vi "control_posicion_DAQ.vi"() -> ()   [LabVIEW 2025]
uses:
  <vilib>/addons/control/pid/pid.llb/PID (DBL).vi
  <vilib>/addons/control/pid/NI_PID_pid.lvlib
panel:
  out "Error":dynamicdata(graph)
  out "flaco deseado":dbl
  out "giro negativo":dynamicdata(graph)
  out "giro positivo":dynamicdata(graph)
  out "angulo deseado":dbl
  in  "stop":bool
  in  "output range":cluster{"output high":dbl, "output low":dbl}={"output high"=100.0, "output low"=-100.0} {"output low" format="%.2f"; "output high" format="%.2f"}
  out "E negativo":bool
  out "E positivo":bool
  out "PID gain":dbl format="%.2f"
  in  "PID gains 4":T1={"proportional gain (Kc)"=1.0, "integral time (Ti, min)"=0.01, "derivative time (Td, min)"=0.0} {"derivative time (Td, min)" format="%.3f"; "integral time (Ti, min)" format="%.3f"; "proportional gain (Kc)" format="%.3f"}
  out "Error":dbl
  in  "valor deseado":dbl(knob) scale=0.0..360.0
  out "Posición (ángulo)":dbl
  out "Posición (flancos)":i32
  out "B":i32
  out "A":i32
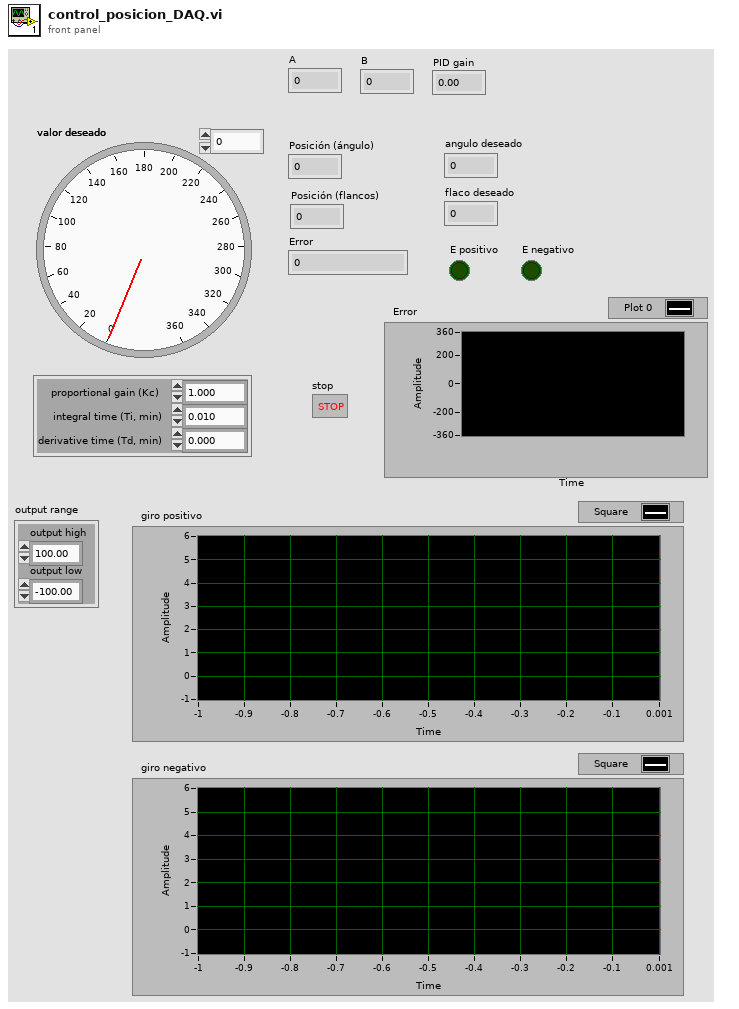
[diagram p1: front panel]
types:
  T1 = cluster{"proportional gain (Kc)":dbl, "integral time (Ti, min)":dbl, "derivative time (Td, min)":dbl}
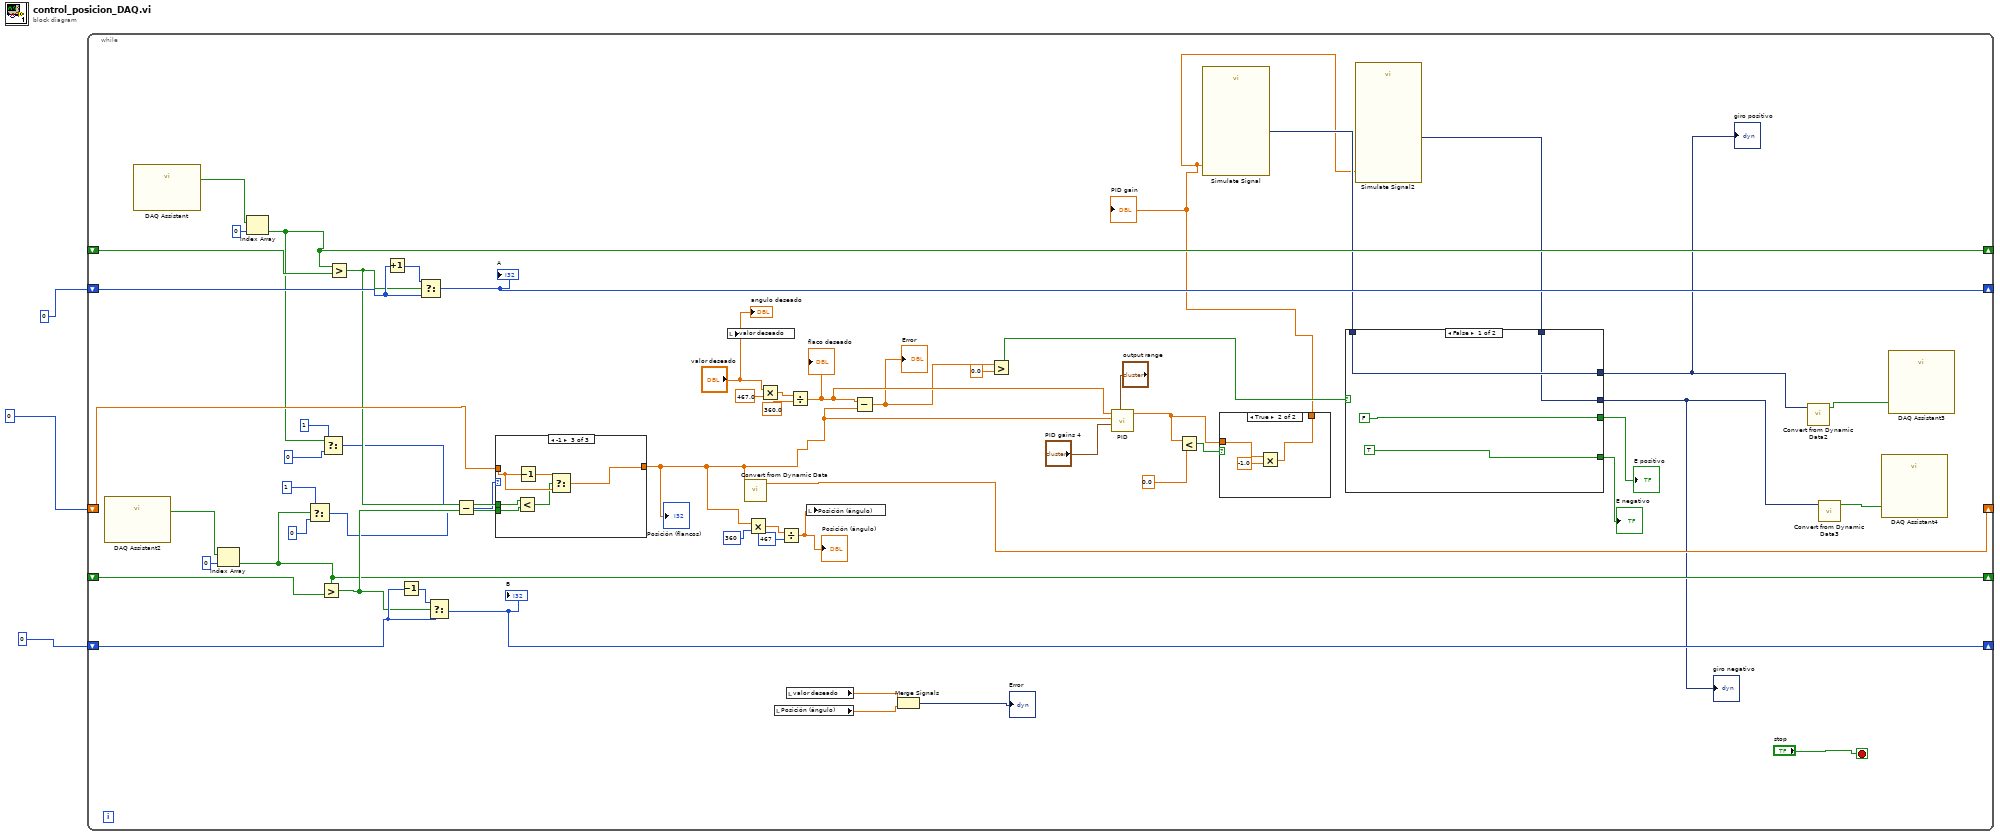
[diagram p0: block diagram]
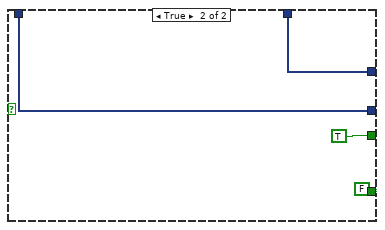
[diagram p3: hidden frame]
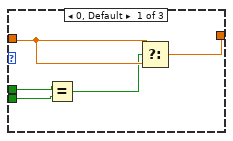
[diagram p4: hidden frame]
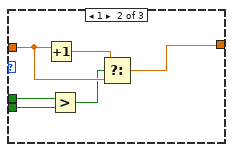
[diagram p5: hidden frame]
diagram:
  n1 = while {
    shift-right: [w45] -> _
    shift-left: _ -> [w59]
    shift-right: [w53] -> _
    shift-left: 0 -> [w57]
    shift-right: [w28] -> _
    shift-left: _ -> [w34]
    shift-right: [w56] -> _
    shift-left: 0 -> [w54]
    shift-right: [w20] -> _
    shift-left: 0 -> [w52]
    stop <- "stop" stop-if-true
    n2 = call "DAQ Assistant2"() -> ("data"=w46:bool[])  [unwired: 17 in, 2 out]
    n3 = call "DAQ Assistant"() -> ("data"=w49:bool[])  [unwired: 17 in, 2 out]
    n4 = Index Array(array=w46, index=0) -> (element=w28:bool)
    n5 = Index Array(array=w49, index=0) -> (element=w45:bool)
    n6 = Select(t=1, s=w28, f=0) -> (s? t:f=w40:i32)
    n7 = Greater?(x=w28, y=w34) -> (0:w50:bool)
    n8 = Select(t=1, s=w45, f=0) -> (s? t:f=w39:i32)
    n9 = Greater?(x=w45, y=w59) -> (0:w51:bool)
    n10 = Increment(x=w57) -> (x+1=w58:i32)
    n11 = Decrement(x=w54) -> (x-1=w55:i32)
    n12 = Select(t=w58, s=w51, f=w57) -> (s? t:f=w53:i32)
    "A" <- w53
    n13 = Select(t=w55, s=w50, f=w54) -> (s? t:f=w56:i32)
    "B" <- w56
    n14 = Subtract(x=w39, y=w40) -> (x-y=w38:i32)
    n15 = case shown="-1" w38 {
      tunnel: w52 -> [w76 w81 w87]
      tunnel: [w75 w80 w86] -> w9
      tunnel: w51 -> [w74 w79 w85]
      tunnel: w50 -> [w73 w78 w84]
      frame 0, Default {
        n16 = Equal?(x=w74, y=w73) -> (x = y?=w72:bool)
        n17 = Select(t=w76, s=w72, f=w76) -> (s? t:f=w75:dbl)
      }
      frame 1 {
        n18 = Increment(x=w81) -> (x+1=w82:dbl)
        n19 = Greater?(x=w79, y=w78) -> (0:w77:bool)
        n20 = Select(t=w82, s=w77, f=w81) -> (s? t:f=w80:dbl)
      }
      frame -1 {
        n21 = Less?(x=w85, y=w84) -> (x < y?=w83:bool)
        n22 = Decrement(x=w87) -> (x-1=w88:dbl)
        n23 = Select(t=w88, s=w83, f=w87) -> (s? t:f=w86:dbl)
      }
    }
    "Posición (flancos)" <- w9
    n24 = local write "valor deseado"("valor deseado") -> ()
    n25 = call "Convert from Dynamic Data"("Dynamic Data Type"=w9) -> ("Scalar"=w20:dbl)  [unwired: 3 in]
    n26 = Multiply(x=w9, y=360) -> (x*y=w35:dbl)
    n27 = Multiply(x="valor deseado", y=467.0) -> (x*y=w32:dbl)
    n28 = local read "Posición (ángulo)"() -> (w5:dbl)
    n29 = Divide(x=w35, y=467) -> (x/y=w6:dbl)
    "Posición (ángulo)" <- w6
    n30 = local read "valor deseado"() -> (w7:dbl)
    n31 = Divide(x=w32, y=360.0) -> (x/y=w16:dbl)
    "flaco deseado" <- w16
    n32 = local write "Posición (ángulo)"(w6) -> ()
    n33 = Subtract(x=w16, y=w9) -> (x-y=w10:dbl)
    "Error" <- w10
    n34 = Merge Signals(w7, w5) -> (→"Error":dynamicdata)
    n35 = Greater?(x=w10, y=0.0) -> (0:w23:bool)
    n36 = call-poly <vilib>:"PID.vi"("output range"="output range", "PID gains"="PID gains 4", "process variable"=w9, "setpoint"=w16) -> ("output"=w11:dbl)  [unwired: 6 in, 1 out]
    n37 = Less?(x=w11, y=0.0 ("x")) -> (x < y?=w14:bool)
    n38 = case shown="True" w14 {
      tunnel: w11 -> [w60 w62]
      tunnel: [w60 w61] -> w13
      frame False {
      }
      frame True {
        n39 = Multiply(x=w62, y=-1.0) -> (x*y=w61:dbl)
      }
    }
    "PID gain" <- w13
    n40 = call "Simulate Signal"("Duty Cycle (%)"=w13) -> ("Square"=w22:dynamicdata)  [unwired: 13 in, 1 out]
    n41 = call "Simulate Signal2"("Duty Cycle (%)"=w13) -> ("Square"=w21:dynamicdata)  [unwired: 13 in, 1 out]
    n42 = case shown="False" w23 {
      tunnel: [FALSE ("E negativo") TRUE ("E positivo")] -> w27
      tunnel: [TRUE ("E negativo") FALSE ("E positivo")] -> w26
      tunnel: [w64 w69] -> w17
      tunnel: w22 -> [w65 w69]
      tunnel: [w65 w68] -> w15
      tunnel: w21 -> [w64 w68]
      frame False {
      }
      frame True {
      }
    }
    "E positivo" <- w27
    "E negativo" <- w26
    "giro positivo" <- w15
    "giro negativo" <- w17
    n43 = call "Convert from Dynamic Data2"("Dynamic Data Type"=w15) -> ("Array"=w19:bool[])  [unwired: 3 in]
    n44 = call "Convert from Dynamic Data3"("Dynamic Data Type"=w17) -> ("Array"=w18:bool[])  [unwired: 3 in]
    n45 = call "DAQ Assistant4"("data"=w18) -> ()  [unwired: 17 in, 2 out]
    n46 = call "DAQ Assistant3"("data"=w19) -> ()  [unwired: 17 in, 2 out]
    "angulo deseado" <- "valor deseado"
  }
